vi "clear_buffers.vi"(8 "error in (no error)":errorcluster, 11 "FPGAWrapperMH120124FrameScan_PXI7813R in":refnum<class "FPGAWrapperMH120124FrameScan_PXI7813R.lvclass">) -> (0 "error out":errorcluster, 3 "FPGAWrapperMH120124FrameScan_PXI7813R out":refnum<class "FPGAWrapperMH120124FrameScan_PXI7813R.lvclass">)   [LabVIEW 2010, in "FPGAWrapperMH120124FrameScan_PXI7813R.lvclass"]
uses:
  FPGAWrapperMH120124FrameScan_PXI7813R.lvclass
  grabber/command_enum.ctl
  class_data.vi
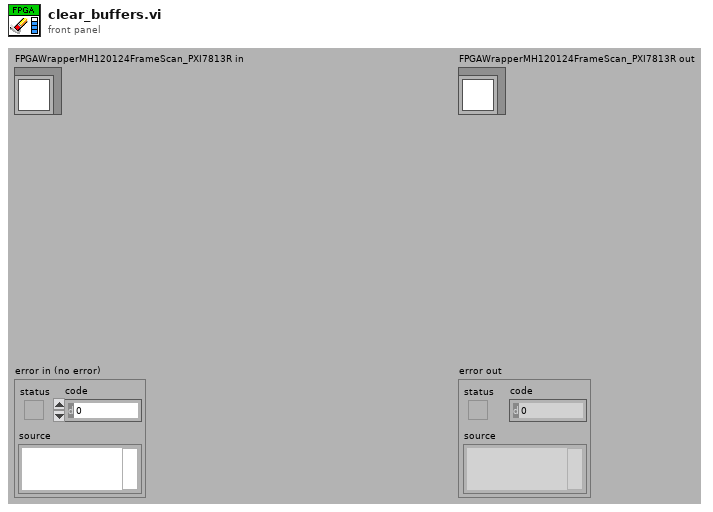
[diagram p1: front panel]
types:
  T1 = typedef "command_enum.ctl" = enum8{"NULL", "update", "start", "stop", "reset", "shut-down"}
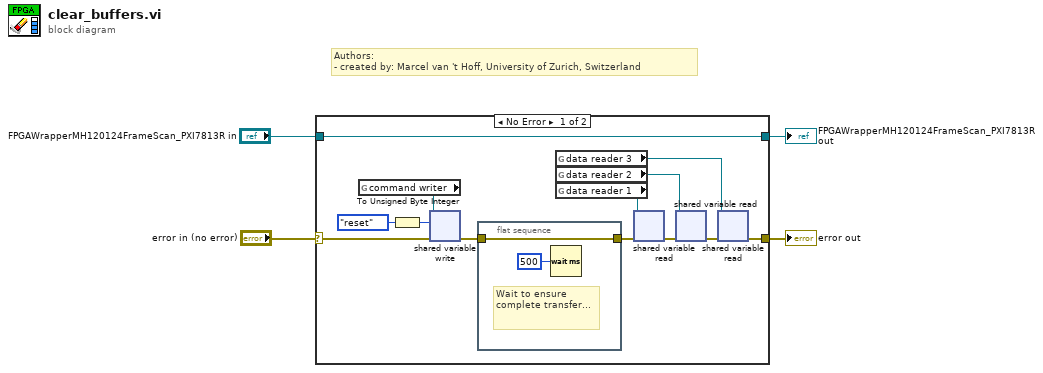
[diagram p0: block diagram]
diagram:
  # "Authors: \n- created by: Marcel van 't Hoff, University of Zurich, Switzerland"
  n1 = case shown="No Error" "error in (no error)" {
    selector: "error in (no error)" -> [w14 w20]
    tunnel: [w10 w20] -> w3
    tunnel: [w17 w21] -> w2
    tunnel: "FPGAWrapperMH120124FrameScan_PXI7813R in" -> [w17 w21]
    frame No Error {
      n2 = global read "class_data.vi" "command writer"() -> (w13:refnum<k21>)
      n3 = To Unsigned Byte Integer(number=command_enum."reset" ("command")) -> (unsigned 8bit integer=w5:u8)
      n4 = shared-variable-write(w13, w14, w5) -> (w15:errorcluster)  [unwired: 1 in, 2 out]
      n5 = flat-sequence {
        tunnel: w15 -> [w19]
        tunnel: [w19] -> w16
        frame #0 {
          # "Wait to ensure complete transfer..."
          n6 = Wait (ms)(milliseconds to wait=u32 500) -> ()  [unwired: 1 out]
        }
      }
      n7 = global read "class_data.vi" "data reader 3"() -> (w7:refnum<k21>)
      n8 = global read "class_data.vi" "data reader 2"() -> (w8:refnum<k21>)
      n9 = global read "class_data.vi" "data reader 1"() -> (w9:refnum<k21>)
      n10 = shared-variable-read(w9, w16) -> (w12:errorcluster)  [unwired: 2 in, 3 out]
      n11 = shared-variable-read(w8, w12) -> (w11:errorcluster)  [unwired: 2 in, 3 out]
      n12 = shared-variable-read(w7, w11) -> (w10:errorcluster)  [unwired: 2 in, 3 out]
    }
    frame Error {
    }
  }
  "error out" <- w3
  "FPGAWrapperMH120124FrameScan_PXI7813R out" <- w2
